vi "Chart.PrepereSamples.vi"(6 "Window Lenght":i32, 8 "Rising?":bool, 9 "Trigger Level":dbl, 10 "Trigger Signal":i32, 11 "Array in":dbl[][](array[numeric])) -> (3 "Array out":dbl[][](array[numeric]))   [LabVIEW 2017, in "Chart.lvlib"]
uses:
  Chart.lvlib
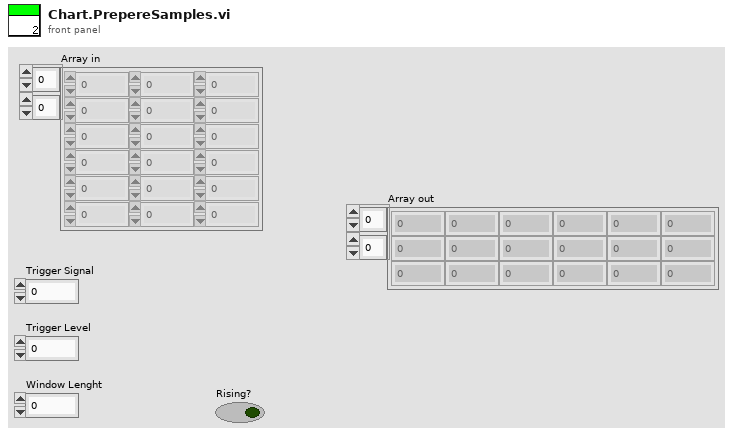
[diagram p1: front panel]
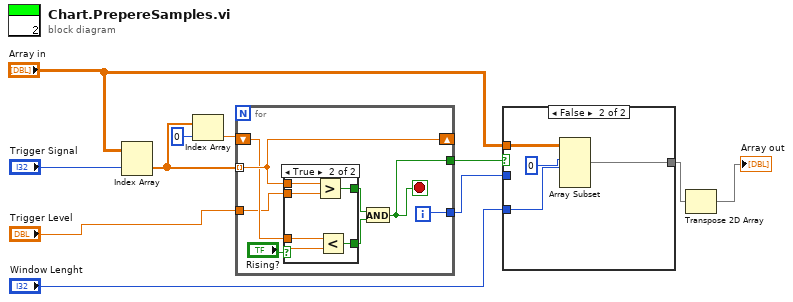
[diagram p0: block diagram]
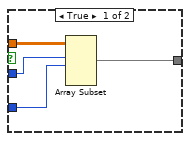
[diagram p2: hidden frame]
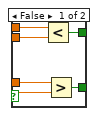
[diagram p3: hidden frame]
diagram:
  n1 = Index Array(array="Array in", index (col)="Trigger Signal") -> (element=w4:dbl[])  [unwired: 1 in]
  n2 = Index Array(array=w4, index=0) -> (element=w2:dbl)
  n3 = for {
    tunnel: w4 -> [w18] mode=indexing
    tunnel: [w13] -> w5
    tunnel: [w19] -> w6
    tunnel: "Trigger Level" -> [w16]
    shift-right: [w18] -> _
    shift-left: w2 -> [w17]
    i -> [w19]
    stop <- w13 stop-if-true
    n4 = case shown="True" "Rising?" {
      tunnel: w18 -> [w24 w29]
      tunnel: w17 -> [w23 w28]
      tunnel: w16 -> [w22 w27]
      tunnel: [w21 w26] -> w15
      tunnel: [w20 w25] -> w14
      frame False {
        n5 = Less?(x=w24, y=w22) -> (x < y?=w21:bool)
        n6 = Greater?(x=w23, y=w22) -> (0:w20:bool)
      }
      frame True {
        n7 = Greater?(x=w29, y=w27) -> (0:w26:bool)
        n8 = Less?(x=w28, y=w27) -> (x < y?=w25:bool)
      }
    }
    n9 = And(x=w15, y=w14) -> (x .and. y?=w13:bool)
  }
  n10 = case shown="False" w5 {
    tunnel: "Array in" -> [w33 w37]
    tunnel: w6 -> [w32 _]
    tunnel: "Window Lenght" -> [w31 w34]
    tunnel: [w30 w36] -> w8
    frame True {
      n11 = Array Subset(array=w33, index (row)=w32, length (row)=w31) -> (w30:dbl[][])  [unwired: 2 in]
    }
    frame False {
      n12 = Array Subset(array=w37, index (row)=0 ("index"), length (row)=w34) -> (w36:dbl[][])  [unwired: 2 in]
    }
  }
  n13 = Transpose 2D Array(2D array=w8) -> (transposed array=→"Array out":dbl[][])
